vi "PCI1220U初始化2.vi"() -> (0 "DevAxesCount":u32, 1 "DeviceNum List":u32[](array[numeric]), 2 "AxisHandle OUT":u32, 3 "DeviceHandle":u32)   [LabVIEW 2013]
panel:
  out "error out 3":errorcluster
  out "error out 2":errorcluster
  out "error out":errorcluster
  out "ReturnValue 4":u32
  out "ReturnValue 3":u32
  out "ReturnValue 2":u32
  out "ReturnValue":u32
  out "Device Type 2":u16(ring) items=["PCI-1240 (M0)"]
  out "AxisOpened":bool
  in  "Device Type":u16(ring) items=["PCI-1240 (M0)"]
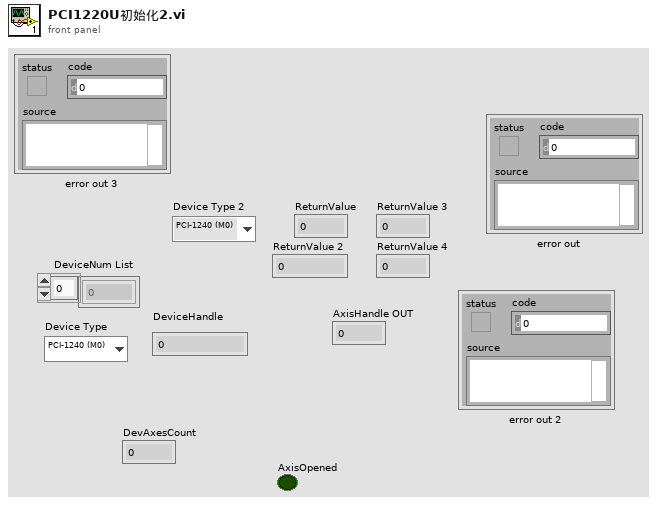
[diagram p1: front panel]
types:
  T1 = cluster{"DeviceNum":u32, "U*8 Array":cluster{"U*8 Array[0]":u8, "U*8 Array[1]":u8, "U*8 Array[2]":u8, "U*8 Array[3]":u8, "U*8 Array[4]":u8, "U*8 Array[5]":u8, "U*8 Array[6]":u8, "U*8 Array[7]":u8, "U*8 Array[8]":u8, "U*8 Array[9]":u8, "U*8 Array[10]":u8, "U*8 Array[11]":u8, "U*8 Array[12]":u8, "U*8 Array[13]":u8, "U*8 Array[14]":u8, "U*8 Array[15]":u8, "U*8 Array[16]":u8, "U*8 Array[17]":u8, "U*8 Array[18]":u8, "U*8 Array[19]":u8, "U*8 Array[20]":u8, "U*8 Array[21]":u8, "U*8 Array[22]":u8, "U*8 Array[23]":u8, "U*8 Array[24]":u8, "U*8 Array[25]":u8, "U*8 Array[26]":u8, "U*8 Array[27]":u8, "U*8 Array[28]":u8, "U*8 Array[29]":u8, "U*8 Array[30]":u8, "U*8 Array[31]":u8, "U*8 Array[32]":u8, "U*8 Array[33]":u8, "U*8 Array[34]":u8, "U*8 Array[35]":u8, "U*8 Array[36]":u8, "U*8 Array[37]":u8, "U*8 Array[38]":u8, "U*8 Array[39]":u8, "U*8 Array[40]":u8, "U*8 Array[41]":u8, "U*8 Array[42]":u8, "U*8 Array[43]":u8, "U*8 Array[44]":u8, "U*8 Array[45]":u8, "U*8 Array[46]":u8, "U*8 Array[47]":u8, "U*8 Array[48]":u8, "U*8 Array[49]":u8}, "NumOfSubDevice":i16}[]
  T2 = cluster{"U*8 Array[0]":u8, "U*8 Array[1]":u8, "U*8 Array[2]":u8, "U*8 Array[3]":u8, "U*8 Array[4]":u8, "U*8 Array[5]":u8, "U*8 Array[6]":u8, "U*8 Array[7]":u8, "U*8 Array[8]":u8, "U*8 Array[9]":u8, "U*8 Array[10]":u8, "U*8 Array[11]":u8, "U*8 Array[12]":u8, "U*8 Array[13]":u8, "U*8 Array[14]":u8, "U*8 Array[15]":u8, "U*8 Array[16]":u8, "U*8 Array[17]":u8, "U*8 Array[18]":u8, "U*8 Array[19]":u8, "U*8 Array[20]":u8, "U*8 Array[21]":u8, "U*8 Array[22]":u8, "U*8 Array[23]":u8, "U*8 Array[24]":u8, "U*8 Array[25]":u8, "U*8 Array[26]":u8, "U*8 Array[27]":u8, "U*8 Array[28]":u8, "U*8 Array[29]":u8, "U*8 Array[30]":u8, "U*8 Array[31]":u8, "U*8 Array[32]":u8, "U*8 Array[33]":u8, "U*8 Array[34]":u8, "U*8 Array[35]":u8, "U*8 Array[36]":u8, "U*8 Array[37]":u8, "U*8 Array[38]":u8, "U*8 Array[39]":u8, "U*8 Array[40]":u8, "U*8 Array[41]":u8, "U*8 Array[42]":u8, "U*8 Array[43]":u8, "U*8 Array[44]":u8, "U*8 Array[45]":u8, "U*8 Array[46]":u8, "U*8 Array[47]":u8, "U*8 Array[48]":u8, "U*8 Array[49]":u8}
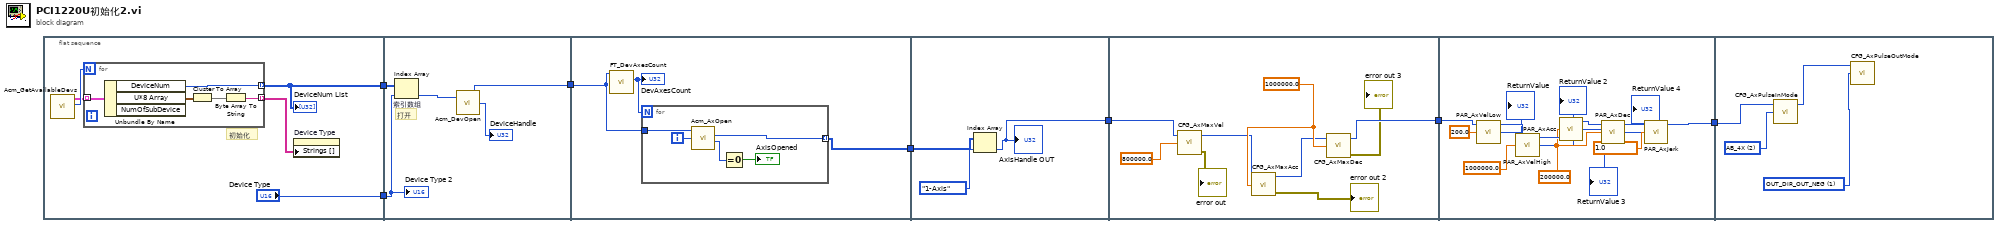
[diagram p0: block diagram]
diagram:
  n1 = flat-sequence {
    tunnel: [w9] -> w7
    tunnel: ["Device Type"] -> w6
    tunnel: w7 -> [w22]
    tunnel: w6 -> [w18]
    tunnel: [w20] -> w5
    tunnel: w5 -> [w24]
    tunnel: [w23] -> w4
    tunnel: w4 -> [w33]
    tunnel: [w31] -> w3
    tunnel: w3 -> [w38]
    tunnel: [w37] -> w2
    tunnel: w2 -> [w56]
    tunnel: [w43] -> w1
    tunnel: w1 -> [w59]
    frame #0 {
      # "初始化"
      n2 = call <userlib>:"Acm_GetAvailableDevs.vi"() -> ("OutEntries"=w12:u32, "DeviceList"=w11:T1)  [unwired: 1 in, 2 out]
      n3 = for {
        N: w12 -> [_]
        tunnel: w11 -> [w17] mode=indexing
        tunnel: [w14] -> w9 mode=indexing
        tunnel: [w13] -> w10 mode=indexing
        n4 = Unbundle By Name(w17) -> ("DeviceNum"=w14:u32, "U*8 Array"=w16:T2)  [unwired: 1 out]
        n5 = Cluster To Array(cluster=w16) -> (array=w15:u8[])
        n6 = Byte Array To String(unsigned byte array=w15) -> (string=w13:string)
      }
      "DeviceNum List" <- w9
      n7 = property on="Device Type" class="Ring (严格)"("Strings []"=w10) -> ()  [unwired: 2 in, 2 out]
    }
    frame #1 {
      # "打开"
      n8 = Index Array "索引数组"(array=w22, index=w18) -> (element=w21:u32)
      n9 = call <userlib>:"Acm_DevOpen.vi"("DeviceNumber"=w21) -> ("ReturnValue"=→"DeviceHandle":u32, "DeviceHandle"=w20:u32)  [unwired: 1 in, 1 out]
      "Device Type 2" <- w18
    }
    frame #2 {
      n10 = call <userlib>:"FT_DevAxesCount.vi"("Handle"=w24) -> ("DevAxesCount"=w25:u32)  [unwired: 3 in, 4 out]
      "DevAxesCount" <- w25
      n11 = for {
        N: w25 -> [_]
        tunnel: w24 -> [w30]
        tunnel: [w26] -> w23 mode=indexing
        i -> [w29]
        n12 = call <userlib>:"Acm_AxOpen.vi"("PhyAxis"=w29, "DeviceHandle"=w30) -> ("ReturnValue"=w28:u32, "AxisHandle"=w26:u32)  [unwired: 1 in, 2 out]
        n13 = Equal To 0?(x=w28) -> (x = 0?=→"AxisOpened":bool)
      }
    }
    frame #3 {
      n14 = Index Array(array=w33, index=enum32{"0-Axis", "1-Axis", "2-Axis", "3-Axis"}."1-Axis" ("Operate Axis")) -> (element=w31:u32)
      "AxisHandle OUT" <- w31
    }
    frame #4 {
      w42 = 1000000.0 ("CFG_AxMaxAcc")
      n15 = call <userlib>:"CFG_AxMaxVel.vi"("CFG_AxMaxVel"=800000.0, "Handle"=w38) -> ("Error Output"=→"error out":errorcluster, "Handle 2"=w40:u32)  [unwired: 1 in, 1 out]
      n16 = call <userlib>:"CFG_AxMaxAcc.vi"("CFG_AxMaxAcc"=w42, "Handle"=w40) -> ("Error Output"=→"error out 2":errorcluster, "Handle 2"=w41:u32)  [unwired: 1 in, 1 out]
      n17 = call <userlib>:"CFG_AxMaxDec.vi"("CFG_AxMaxDec"=w42, "Handle"=w41) -> ("Error Output"=→"error out 3":errorcluster, "Handle 2"=w37:u32)  [unwired: 1 in, 1 out]
    }
    frame #5 {
      w48 = 1.0 items=["T-curve", "S-curve"] ("PAR_AxJerk")
      w49 = 200000.0 ("PAR_AxAcc")
      n18 = call <userlib>:"PAR_AxVelLow.vi"("PAR_AxVelLow"=200.0, "Handle"=w56) -> ("ReturnValue"=→"ReturnValue":u32, "Handle 2"=w55:u32)  [unwired: 1 in, 1 out]
      n19 = call <userlib>:"PAR_AxVelHigh.vi"("PAR_AxVelHigh"=1000000.0, "Handle"=w55) -> ("ReturnValue"=→"ReturnValue 2":u32, "Handle 2"=w54:u32)  [unwired: 1 in, 1 out]
      n20 = call <userlib>:"PAR_AxAcc.vi"("PAR_AxAcc"=w49, "Handle"=w54) -> ("ReturnValue"=→"ReturnValue 3":u32, "Handle 2"=w53:u32)  [unwired: 1 in, 1 out]
      n21 = call <userlib>:"PAR_AxDec.vi"("PAR_AxDec"=w49, "Handle"=w53) -> ("ReturnValue"=→"ReturnValue 4":u32, "Handle 2"=w52:u32)  [unwired: 1 in, 1 out]
      n22 = call <userlib>:"PAR_AxJerk.vi"("PAR_AxJerk"=w48, "Handle"=w52) -> ("Handle 2"=w43:u32)  [unwired: 1 in, 2 out]
    }
    frame #6 {
      w57 = u32 2 items=["AB_1X", "AB_2X", "AB_4X", "I_CW_CCW"] ("CFG_AxPulseInMode")
      w58 = u32 1 items=["OUT_DIR", "OUT_DIR_OUT_NEG", "OUT_DIR_DIR_NEG", "OUT_DIR_ALL_NEG", "O_CW_CCW", "CW_CCW_ALL_NEG", "AB_PHASE", "BA_PHASE", "CW_CCW_OUT_NEG", "CW_CCW_DIR_NEG"] ("CFG_AxPulseOutMode")
      n23 = call <userlib>:"CFG_AxPulseInMode.vi"("CFG_AxPulseInMode"=w57, "Handle"=w59) -> ("Handle 2"=w60:u32)  [unwired: 1 in, 2 out]
      n24 = call <userlib>:"CFG_AxPulseOutMode.vi"("CFG_AxPulseOutMode"=w58, "Handle"=w60) -> ()  [unwired: 1 in, 3 out]
    }
  }
